vi "LV homework #5 sub-VI.vi"(11 "Numeric Input":dbl) -> (3 "Results":dbl[](array[numeric]))   [LabVIEW 2018]
panel:
  out "Results copy":dbl[](array[numeric])
  # "I changed this from x^2 & sqrt(x) to (x+2) & (x-2)"
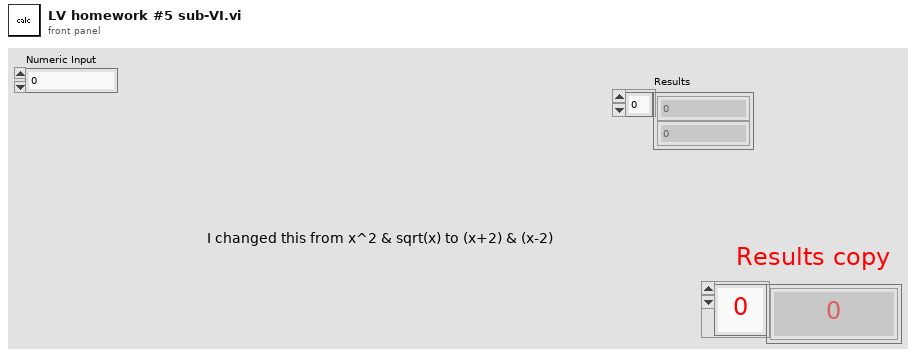
[diagram p1: front panel]
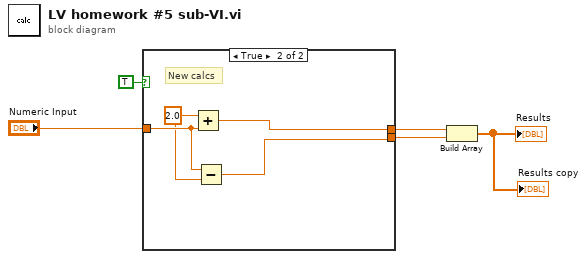
[diagram p0: block diagram]
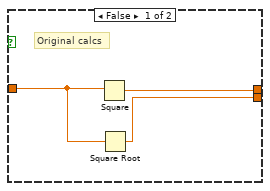
[diagram p2: hidden frame]
diagram:
  n1 = case shown="True" TRUE {
    tunnel: "Numeric Input" -> [w8 w12]
    tunnel: [w7 w10] -> w4
    tunnel: [w6 w9] -> w3
    frame False {
      # "Original calcs"
      n2 = Square(x=w8) -> (x^2=w7:dbl)
      n3 = Square Root(x=w8) -> (sqrt(x)=w6:dbl)
    }
    frame True {
      w11 = 2.0 ("x")
      # "New calcs"
      n4 = Add(x=w11, y=w12) -> (x+y=w10:dbl)
      n5 = Subtract(x=w12, y=w11) -> (x-y=w9:dbl)
    }
  }
  n6 = Build Array(w4, w3) -> (→"Results" →"Results copy":dbl[])
